vi "IRSensor(SubVI).vi"(11 "Array":dbl[](array[numeric])) -> (3 "interpolation value":dbl)   [LabVIEW 2017]
uses:
  <vilib>/Analysis/baseanly.llb/Mean (DBL).vi
  <vilib>/Analysis/NI_AALPro.lvlib
  <vilib>/Analysis/NI_AALBase.lvlib
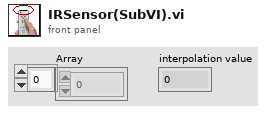
[diagram p1: front panel]
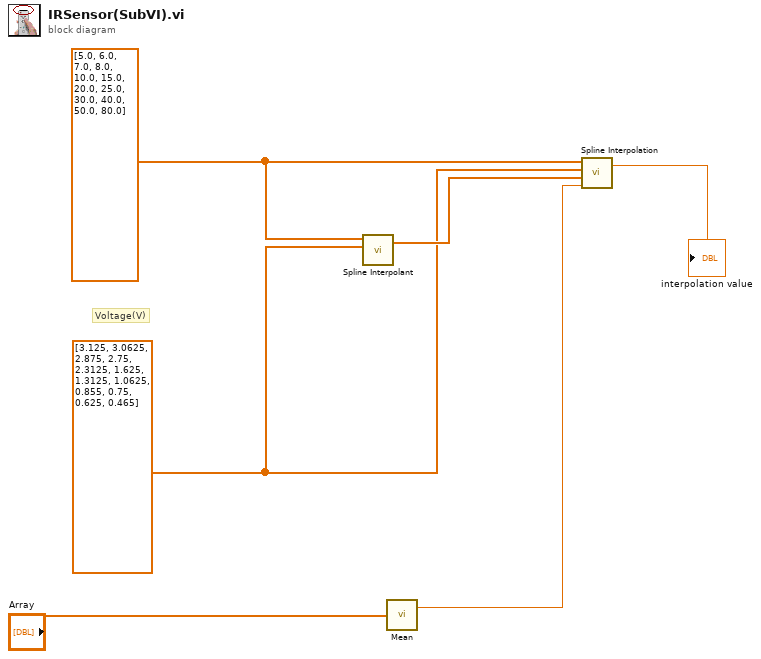
[diagram p0: block diagram]
diagram:
  w1 = dbl[] [5.0, 6.0, 7.0, 8.0, 10.0, 15.0, 20.0, 25.0, 30.0, 40.0, 50.0, 80.0]
  w2 = dbl[] [3.125, 3.0625, 2.875, 2.75, 2.3125, 1.625, 1.3125, 1.0625, 0.855, 0.75, 0.625, 0.465]
  # "Voltage(V)"
  n1 = call <vilib>:"Spline Interpolant.vi"("X"=w2, "Y"=w1) -> ("Interpolant"=w3:dbl[])  [unwired: 2 in, 1 out]
  n2 = call-poly <vilib>:"Mean.vi"("X"="Array") -> ("mean"=w4:dbl)  [unwired: 1 out]
  n3 = call <vilib>:"Spline Interpolation.vi"("x value"=w4, "Interpolant"=w3, "X"=w2, "Y"=w1) -> ("interpolation value"=→"interpolation value":dbl)  [unwired: 1 out]
